vi "Read Measurement Format.vi"(7 "Unit ID (A)":string="A", 8 "error in":errorcluster, 11 "VISA Session In":refnum<visa-resource-name>="Alicat") -> (0 "error out":errorcluster, 2 "Data Frame Format":T1, 3 "VISA Session Out":refnum<visa-resource-name>)   [LabVIEW 2016]
doc: "Determines the format of the data frame. This VI is required for the Read Measurements VI to know how to parse the data properly."
uses:
  <vilib>/Instr/_visa.llb/VISA Flush IO Buffer Mask.ctl
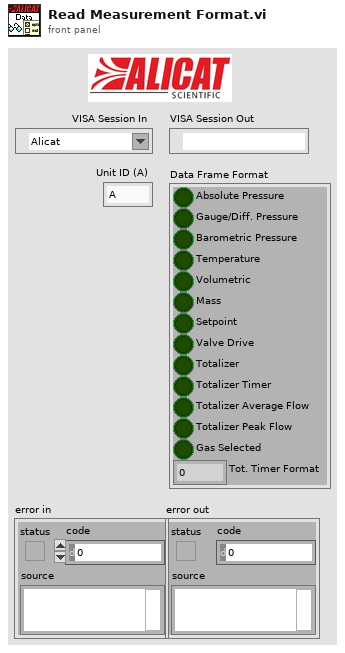
[diagram p1: front panel]
types:
  T1 = cluster{"Absolute Pressure":bool, "Gauge/Diff. Pressure":bool, "Barometric Pressure":bool, "Temperature":bool, "Volumetric":bool, "Mass":bool, "Setpoint":bool, "Valve Drive":bool, "Totalizer":bool, "Totalizer Timer":bool, "Totalizer Average Flow":bool, "Totalizer Peak Flow":bool, "Gas Selected":bool, "Tot. Timer Format":u16}
  T2 = typedef "VISA Flush IO Buffer Mask.ctl" = u16
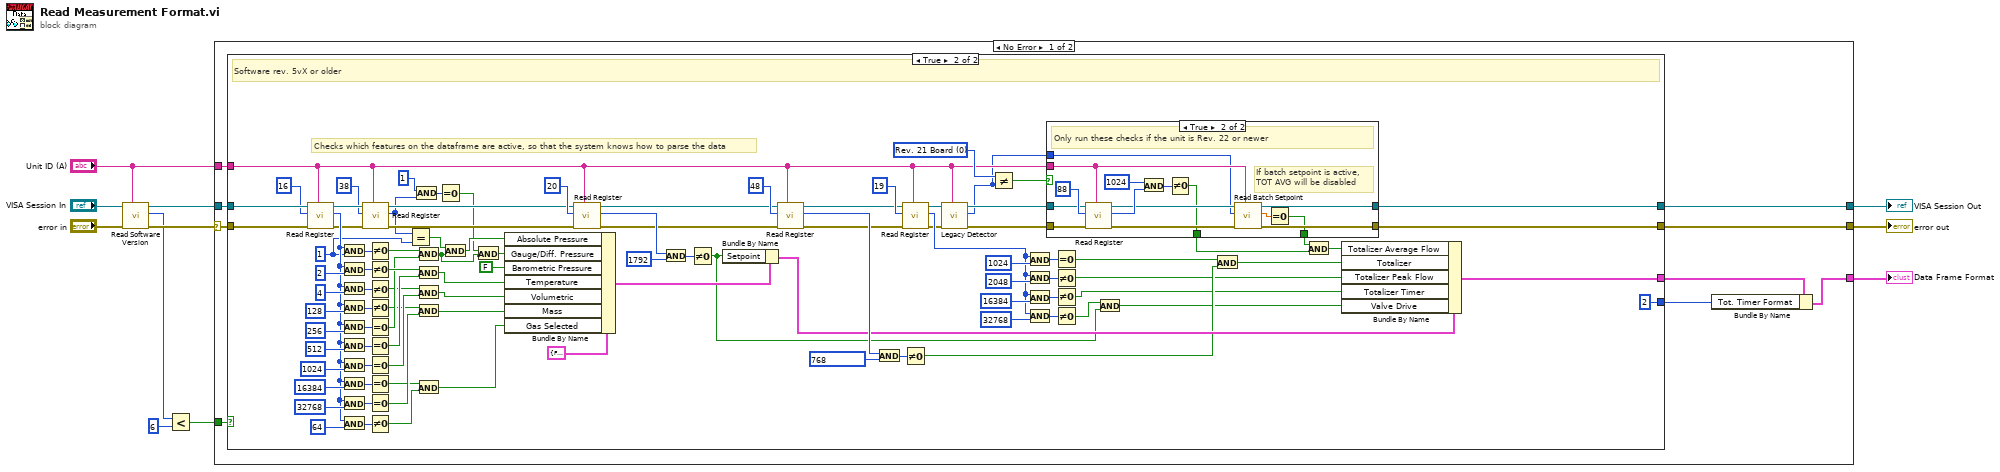
[diagram p0: block diagram]
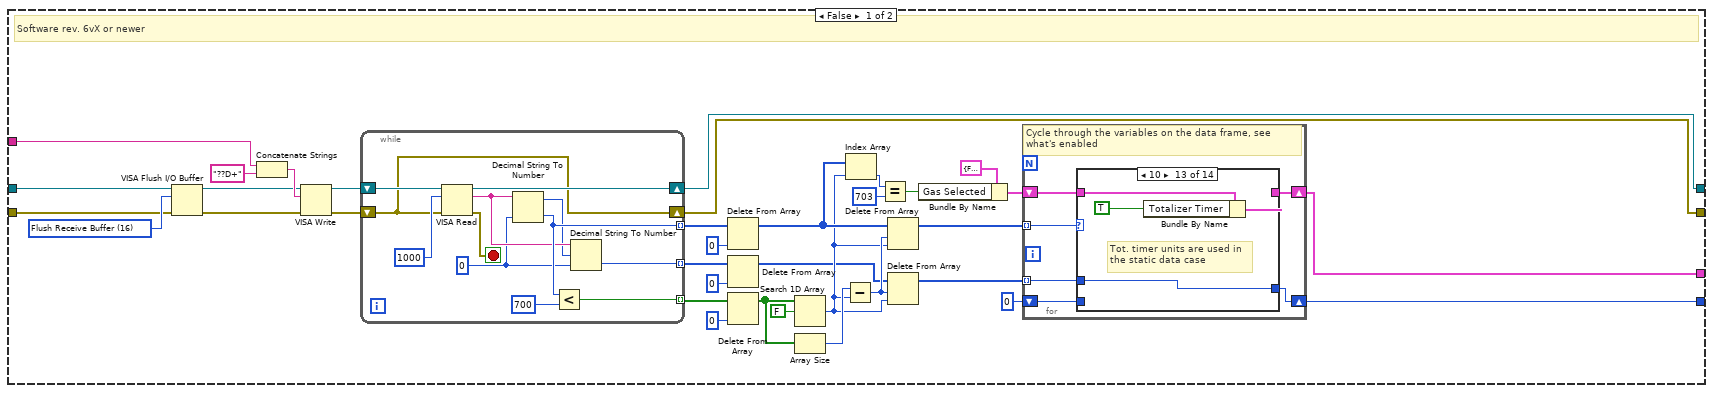
[diagram p2: hidden frame]
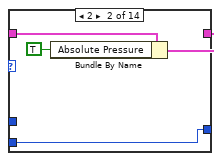
[diagram p4: hidden frame]
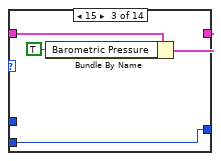
[diagram p5: hidden frame]
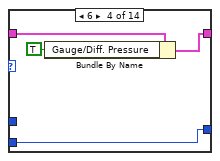
[diagram p6: hidden frame]
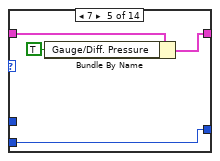
[diagram p7: hidden frame]
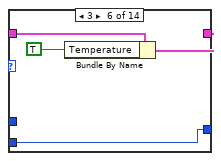
[diagram p8: hidden frame]
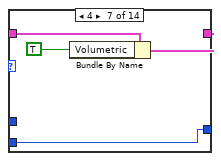
[diagram p9: hidden frame]
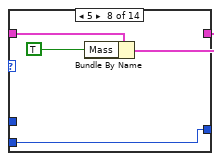
[diagram p10: hidden frame]
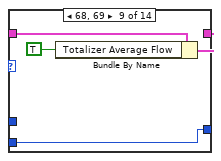
[diagram p11: hidden frame]
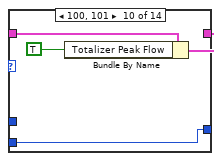
[diagram p12: hidden frame]
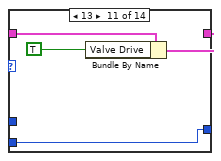
[diagram p13: hidden frame]
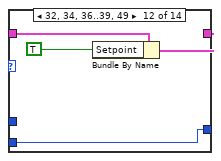
[diagram p14: hidden frame]
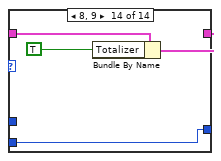
[diagram p15: hidden frame]
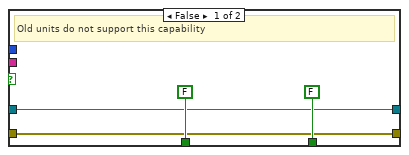
[diagram p16: hidden frame]
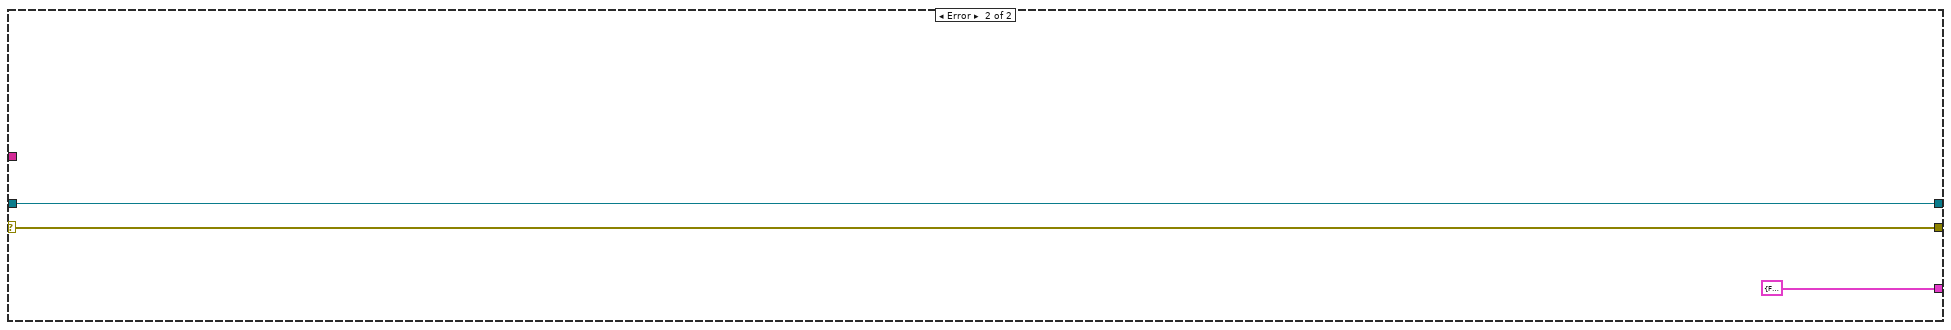
[diagram p17: hidden frame]
diagram:
  n1 = call "Read Software Version.vi"("Unit ID (A)"="Unit ID (A)", "error in"="error in", "VISA Session In"="VISA Session In") -> ("error out"=w4:errorcluster, "Software Version"=w2:u8, "VISA Session Out"=w3:refnum<visa-resource-name>)  [unwired: 6 in]
  n2 = Less?(x=w2, y=u8 6) -> (x < y?=w8:bool)
  n3 = case shown="No Error" w4 {
    selector: w4 -> [w19 w248]
    tunnel: w3 -> [w20 w249]
    tunnel: "Unit ID (A)" -> [w16 _]
    tunnel: [w12 T1 {"Absolute Pressure"=FALSE, "Gauge/Diff. Pressure"=FALSE, "Barometric Pressure"=FALSE, "Temperature"=FALSE, "Volumetric"=FALSE, "Mass"=FALSE, "Setpoint"=FALSE, "Valve Drive"=FALSE, "Totalizer"=FALSE, "Totalizer Timer"=FALSE, "Totalizer Average Flow"=FALSE, "Totalizer Peak Flow"=FALSE, "Gas Selected"=FALSE, "Tot. Timer Format"=0} ("Data Frame Format")] -> w1
    tunnel: [w17 w249] -> w11
    tunnel: [w18 w248] -> w10
    tunnel: w8 -> [w15 _]
    frame No Error {
      n4 = case shown="True" w15 {
        tunnel: w20 -> [w41 w227]
        tunnel: [w33 w168] -> w13
        tunnel: w19 -> [w42 w167]
        tunnel: [w32 w166] -> w18
        tunnel: [w31 w165] -> w17
        tunnel: w16 -> [w40 w142]
        tunnel: [w22 u16 2] -> w14
        frame False {
          w43 = T2 16 items=["Flush Receive Buffer"=16, "Write Transmit Buffer to Device"=32, "Flush Receive Buffer (No I/O)"=64, "Flush Transmit Buffer"=128] ("Mask")
          # "Software rev. 6vX or newer"
          n5 = VISA Flush I/O Buffer(VISA resource name=w41, mask (16)=w43, error in (no error)=w42) -> (VISA resource name out=w44:refnum<visa-resource-name>, error out=w45:errorcluster)
          n6 = Concatenate Strings(w40, "??D+" ("string")) -> (w47:string)
          n7 = VISA Write(VISA resource name=w44, write buffer=w47, error in (no error)=w45) -> (VISA resource name out=w55:refnum<visa-resource-name>, error out=w54:errorcluster)  [unwired: 1 out]
          n8 = while {
            shift-right: [w125] -> w31
            shift-left: w55 -> [w126]
            shift-right: [w124] -> w32
            shift-left: w54 -> [w124]
            tunnel: [w123] -> w51 mode=indexing
            tunnel: [w121] -> w52 mode=indexing
            tunnel: [w116] -> w28 mode=indexing
            stop <- w122 stop-if-true
            w117 = u16 0 ("default value 2")
            n9 = VISA Read(VISA resource name=w126, byte count=u32 1000, error in (no error)=w124) -> (VISA resource name out=w125:refnum<visa-resource-name>, read buffer=w119:string, error out=w122:errorcluster)  [unwired: 1 out]
            n10 = Decimal String To Number(string=w119, default (0L)=w117) -> (offset past number=w118:i32, number=w121:u16)  [unwired: 1 in]
            n11 = Less?(x=w121, y=u16 700) -> (x < y?=w123:bool)
            n12 = Decimal String To Number(string=w119, offset=w118, default (0L)=w117) -> (number=w116:u16)  [unwired: 1 out]
          }
          n13 = Delete From Array(array=w52, index=0) -> (array with subset deleted=w39:u16[])  [unwired: 1 in, 1 out]
          n14 = Delete From Array(array=w28, index=0) -> (array with subset deleted=w25:u16[])  [unwired: 1 in, 1 out]
          n15 = Delete From Array(array=w51, index=0) -> (array with subset deleted=w53:bool[])  [unwired: 1 in, 1 out]
          n16 = Search 1D Array(1D array=w53, element=FALSE) -> (index of element=w26:i32)  [unwired: 1 in]
          n17 = Array Size(array=w53) -> (size(s)=w49:i32)
          n18 = Subtract(x=w49, y=w26) -> (x-y=w27:i32)
          n19 = Index Array(array=w39, index=w26) -> (element=w38:u16)
          n20 = Equal?(x=w38, y=u16 703) -> (x = y?=w36:bool)
          n21 = Delete From Array(array=w39, length=w27, index=w26) -> (array with subset deleted=w34:u16[])  [unwired: 1 out]
          n22 = Delete From Array(array=w25, length=w27, index=w26) -> (array with subset deleted=w24:u16[])  [unwired: 1 out]
          n23 = Bundle By Name(cluster=T1 {"Absolute Pressure"=FALSE, "Gauge/Diff. Pressure"=FALSE, "Barometric Pressure"=FALSE, "Temperature"=FALSE, "Volumetric"=FALSE, "Mass"=FALSE, "Setpoint"=FALSE, "Valve Drive"=FALSE, "Totalizer"=FALSE, "Totalizer Timer"=FALSE, "Totalizer Average Flow"=FALSE, "Totalizer Peak Flow"=FALSE, "Gas Selected"=FALSE, "Tot. Timer Format"=0} ("Data Frame Format"), "Gas Selected"=w36) -> (w35:T1)
          n24 = for {
            tunnel: w34 -> [w61] mode=indexing
            shift-right: [w59] -> w33
            shift-left: w35 -> [w60]
            tunnel: w24 -> [w58] mode=indexing
            shift-right: [w57] -> w22
            shift-left: u16 0 -> [w56]
            # "Cycle through the variables on the data frame, see what's enabled"
            n25 = case shown="10" w61 {
              tunnel: w60 -> [w63 w67 w71 w75 w79 w83 w87 w91 w95 w99 w103 w107 w111 w115]
              tunnel: [w63 w65 w69 w73 w77 w81 w85 w89 w93 w97 w101 w105 w109 w113] -> w59
              tunnel: w58 -> [_ _ _ _ _ _ _ _ _ _ _ _ w108 _]
              tunnel: [w62 w64 w68 w72 w76 w80 w84 w88 w92 w96 w100 w104 w108 w112] -> w57
              tunnel: w56 -> [w62 w64 w68 w72 w76 w80 w84 w88 w92 w96 w100 w104 _ w112]
              frame 0, Default {
              }
              frame 2 {
                n26 = Bundle By Name(cluster=w67, "Absolute Pressure"=TRUE) -> (w65:T1)
              }
              frame 15 {
                n27 = Bundle By Name(cluster=w71, "Barometric Pressure"=TRUE ("Absolute Pressure")) -> (w69:T1)
              }
              frame 6 {
                n28 = Bundle By Name(cluster=w75, "Gauge/Diff. Pressure"=TRUE ("Absolute Pressure")) -> (w73:T1)
              }
              frame 7 {
                n29 = Bundle By Name(cluster=w79, "Gauge/Diff. Pressure"=TRUE ("Absolute Pressure")) -> (w77:T1)
              }
              frame 3 {
                n30 = Bundle By Name(cluster=w83, "Temperature"=TRUE ("Absolute Pressure")) -> (w81:T1)
              }
              frame 4 {
                n31 = Bundle By Name(cluster=w87, "Volumetric"=TRUE ("Absolute Pressure")) -> (w85:T1)
              }
              frame 5 {
                n32 = Bundle By Name(cluster=w91, "Mass"=TRUE ("Absolute Pressure")) -> (w89:T1)
              }
              frame 68, 69 {
                n33 = Bundle By Name(cluster=w95, "Totalizer Average Flow"=TRUE ("Absolute Pressure")) -> (w93:T1)
              }
              frame 100, 101 {
                n34 = Bundle By Name(cluster=w99, "Totalizer Peak Flow"=TRUE ("Absolute Pressure")) -> (w97:T1)
              }
              frame 13 {
                n35 = Bundle By Name(cluster=w103, "Valve Drive"=TRUE ("Absolute Pressure")) -> (w101:T1)
              }
              frame 32, 34, 36..39, 49 {
                n36 = Bundle By Name(cluster=w107, "Setpoint"=TRUE ("Absolute Pressure")) -> (w105:T1)
              }
              frame 10 {
                # "Tot. timer units are used in\nthe static data case"
                n37 = Bundle By Name(cluster=w111, "Totalizer Timer"=TRUE ("Absolute Pressure")) -> (w109:T1)
              }
              frame 8, 9 {
                n38 = Bundle By Name(cluster=w115, "Totalizer"=TRUE ("Absolute Pressure")) -> (w113:T1)
              }
            }
          }
        }
        frame True {
          w156 = u8 0 items=["Rev. 21 Board", "Rev. 22 Board", "Rev. 23 Board"] ("Legacy Status")
          w131 = 1 ("Register Value (U16)")
          # "Checks which features on the dataframe are active, so that the system knows how to parse the data"
          # "Software rev. 5vX or older"
          n39 = call "Read Register.vi"("Unit ID (A)"=w142, "error in"=w167, "Register address"=u16 16, "VISA Session In"=w227) -> ("error out"=w145:errorcluster, "Register Value (I32)"=w154:i32, "VISA Session Out"=w146:refnum<visa-resource-name>)  [unwired: 5 in]
          n40 = And(x=w154, y=w131) -> (x .and. y?=w217:i32)
          n41 = And(x=w154, y=2 ("Register Value (U16)")) -> (x .and. y?=w216:i32)
          n42 = And(x=w154, y=4 ("Register Value (U16)")) -> (x .and. y?=w215:i32)
          n43 = And(x=w154, y=128 ("Register Value (U16)")) -> (x .and. y?=w214:i32)
          n44 = And(x=w154, y=256 ("Register Value (U16)")) -> (x .and. y?=w213:i32)
          n45 = And(x=w154, y=512 ("Register Value (U16)")) -> (x .and. y?=w212:i32)
          n46 = And(x=w154, y=1024 ("Register Value (U16)")) -> (x .and. y?=w211:i32)
          n47 = And(x=w154, y=16384 ("Register Value (U16)")) -> (x .and. y?=w210:i32)
          n48 = And(x=w154, y=32768 ("Register Value (U16)")) -> (x .and. y?=w209:i32)
          n49 = And(x=w154, y=64 ("Register Value (U16)")) -> (x .and. y?=w153:i32)
          n50 = call "Read Register.vi"("Unit ID (A)"=w142, "error in"=w145, "Register address"=u16 38, "VISA Session In"=w146) -> ("error out"=w144:errorcluster, "Register Value (I32)"=w132:i32, "VISA Session Out"=w143:refnum<visa-resource-name>)  [unwired: 5 in]
          n51 = Not Equal To 0?(x=w217) -> (x != 0?=w208:bool)
          n52 = Not Equal To 0?(x=w216) -> (x != 0?=w207:bool)
          n53 = Not Equal To 0?(x=w215) -> (x != 0?=w204:bool)
          n54 = Not Equal To 0?(x=w214) -> (x != 0?=w202:bool)
          n55 = Equal To 0?(x=w213) -> (x = 0?=w206:bool)
          n56 = Equal To 0?(x=w212) -> (x = 0?=w205:bool)
          n57 = Equal To 0?(x=w211) -> (x = 0?=w203:bool)
          n58 = Equal To 0?(x=w210) -> (x = 0?=w152:bool)
          n59 = Equal To 0?(x=w209) -> (x = 0?=w201:bool)
          n60 = Not Equal To 0?(x=w153) -> (x != 0?=w151:bool)
          n61 = Equal?(x=w132, y=w131) -> (x = y?=w133:bool)
          n62 = And(x=1, y=w132) -> (x .and. y?=w138:i32)
          n63 = And(x=w208, y=w206) -> (x .and. y?=w134:bool)
          n64 = And(x=w207, y=w205) -> (x .and. y?=w200:bool)
          n65 = And(x=w204, y=w203) -> (x .and. y?=w199:bool)
          n66 = And(x=w202, y=w201) -> (x .and. y?=w198:bool)
          n67 = And(x=w152, y=w151) -> (x .and. y?=w150:bool)
          n68 = Equal To 0?(x=w138) -> (x = 0?=w135:bool)
          n69 = And(x=w133, y=w134) -> (x .and. y?=w137:bool)
          n70 = And(x=w135, y=w134) -> (x .and. y?=w136:bool)
          n71 = Bundle By Name(cluster=T1 {"Absolute Pressure"=FALSE, "Gauge/Diff. Pressure"=FALSE, "Barometric Pressure"=FALSE, "Temperature"=FALSE, "Volumetric"=FALSE, "Mass"=FALSE, "Setpoint"=FALSE, "Valve Drive"=FALSE, "Totalizer"=FALSE, "Totalizer Timer"=FALSE, "Totalizer Average Flow"=FALSE, "Totalizer Peak Flow"=FALSE, "Gas Selected"=FALSE, "Tot. Timer Format"=0} ("Data Frame Format"), "Absolute Pressure"=w137, "Gauge/Diff. Pressure"=w136, "Barometric Pressure"=FALSE, "Temperature"=w200, "Volumetric"=w199, "Mass"=w198, "Gas Selected"=w150) -> (w187:T1)
          n72 = call "Read Register.vi"("Unit ID (A)"=w142, "error in"=w144, "Register address"=u16 20, "VISA Session In"=w143) -> ("error out"=w181:errorcluster, "Register Value (I32)"=w190:i32, "VISA Session Out"=w182:refnum<visa-resource-name>)  [unwired: 5 in]
          n73 = And(x=w190, y=1792) -> (x .and. y?=w188:i32)
          n74 = Not Equal To 0?(x=w188) -> (x != 0?=w147:bool)
          n75 = Bundle By Name(cluster=w187, "Setpoint"=w147) -> (w178:T1)
          n76 = call "Read Register.vi"("Unit ID (A)"=w142, "error in"=w181, "Register address"=u16 48, "VISA Session In"=w182) -> ("error out"=w180:errorcluster, "Register Value (I32)"=w184:i32, "VISA Session Out"=w179:refnum<visa-resource-name>)  [unwired: 5 in]
          n77 = And(x=w184, y=768) -> (x .and. y?=w186:i32)
          n78 = call "Read Register.vi"("Unit ID (A)"=w142, "error in"=w180, "Register address"=u16 19, "VISA Session In"=w179) -> ("error out"=w160:errorcluster, "Register Value (I32)"=w192:i32, "VISA Session Out"=w161:refnum<visa-resource-name>)  [unwired: 5 in]
          n79 = Not Equal To 0?(x=w186) -> (x != 0?=w172:bool)
          n80 = call "Legacy Detector.vi"("Unit ID (A)"=w142, "error in"=w160, "VISA Session In"=w161) -> ("error out"=w159:errorcluster, "Legacy Status"=w128:u8, "VISA Session Out"=w158:refnum<visa-resource-name>)  [unwired: 6 in]
          n81 = Not Equal?(x=w156, y=w128) -> (x != y?=w157:bool)
          n82 = And(x=w192, y=1024 ("Register Value (U16)")) -> (x .and. y?=w177:i32)
          n83 = And(x=w192, y=2048 ("Register Value (U16)")) -> (x .and. y?=w174:i32)
          n84 = And(x=w192, y=16384 ("Register Value (U16)")) -> (x .and. y?=w176:i32)
          n85 = And(x=w192, y=32768 ("Register Value (U16)")) -> (x .and. y?=w175:i32)
          n86 = case shown="True" w157 {
            tunnel: w158 -> [w229 w245]
            tunnel: w159 -> [w228 w244]
            tunnel: w142 -> [_ w240]
            tunnel: [w228 w238] -> w166
            tunnel: [w229 w236] -> w165
            tunnel: [FALSE w234] -> w163
            tunnel: [FALSE w233] -> w162
            tunnel: w128 -> [_ w232]
            frame False {
              # "Old units do not support this capability"
            }
            frame True {
              # "If batch setpoint is active, \nTOT AVG will be disabled"
              # "Only run these checks if the unit is Rev. 22 or newer"
              n87 = call "Read Register.vi"("Unit ID (A)"=w240, "error in"=w244, "Register address"=u16 88, "VISA Session In"=w245) -> ("error out"=w239:errorcluster, "Register Value (I32)"=w241:i32, "VISA Session Out"=w237:refnum<visa-resource-name>)  [unwired: 5 in]
              n88 = And(x=1024 ("y"), y=w241) -> (x .and. y?=w242:i32)
              n89 = Not Equal To 0?(x=w242) -> (x != 0?=w233:bool)
              n90 = call "Read Batch Setpoint.vi"("Unit ID (A)"=w240, "error in"=w239, "Legacy Status"=w232, "VISA Session In"=w237) -> ("error out"=w238:errorcluster, "Register 92 Value (DBL)"=w235:dbl, "VISA Session Out"=w236:refnum<visa-resource-name>)  [unwired: 5 in]
              n91 = Equal To 0?(x=w235) -> (x = 0?=w234:bool)
            }
          }
          n92 = Equal To 0?(x=w177) -> (x = 0?=w173:bool)
          n93 = Not Equal To 0?(x=w174) -> (x != 0?=w170:bool)
          n94 = Not Equal To 0?(x=w176) -> (x != 0?=w169:bool)
          n95 = Not Equal To 0?(x=w175) -> (x != 0?=w149:bool)
          n96 = And(x=w149, y=w147) -> (x .and. y?=w148:bool)
          n97 = And(x=w173, y=w172) -> (x .and. y?=w171:bool)
          n98 = And(x=w163, y=w162) -> (x .and. y?=w164:bool)
          n99 = Bundle By Name(cluster=w178, "Totalizer Average Flow"=w164, "Totalizer"=w171, "Totalizer Peak Flow"=w170, "Totalizer Timer"=w169, "Valve Drive"=w148) -> (w168:T1)
        }
      }
      n100 = Bundle By Name(cluster=w13, "Tot. Timer Format"=w14) -> (w12:T1)
    }
    frame Error {
    }
  }
  "error out" <- w10
  "VISA Session Out" <- w11
  "Data Frame Format" <- w1
